vi "play-with-variants.vi"() -> ()   [LabVIEW 2019]
uses:
  <vilib>/Utility/Data Type/Type Definitions/Data Type.ctl
  <vilib>/Utility/Data Type/Type Definitions/Type Definition Info.ctl
  <vilib>/Rock Robotics/WPI/ThirdParty/JAS_Junk/TrajLib/SIMPLE_MOTOR_FF.ctl
  <vilib>/Rock Robotics/WPI/ThirdParty/JAS_Junk/TrajLib/MECA_DRIVE_KINEMATICS.ctl
  <vilib>/Rock Robotics/WPI/ThirdParty/JAS_Junk/TrajLib/TRANSLATION2D.ctl
  <vilib>/Analysis/Matrix/Datatypes/RealMatrix.ctl
  <vilib>/Rock Robotics/WPI/ThirdParty/JAS_Junk/TrajLib/SWERVE_DRIVE_KINEMATICS.ctl
  <vilib>/Rock Robotics/SystemInterfaces/NetworkCommunication/NetComm_UsageReport_report.vi
  <vilib>/Rock Robotics/WPI/ThirdParty/JAS_Junk/TrajLib/Util_LibraryGlobals.vi
  <vilib>/Rock Robotics/WPI/ThirdParty/JAS_Junk/TrajLib/Trajectory_Library.lvlib
  <vilib>/Analysis/Matrix/NI_Matrix.lvlib
  <vilib>/Utility/Data Type/NI_Data Type.lvlib
panel:
  out "TypeDefInfo":T1[](array[typedef])
  out "TypeDef":bool[](array[boolean])
  out "Name":string[](array[string])
  out "Type":T2[](array[typedef])
  out "output array":variant[](array[variant])
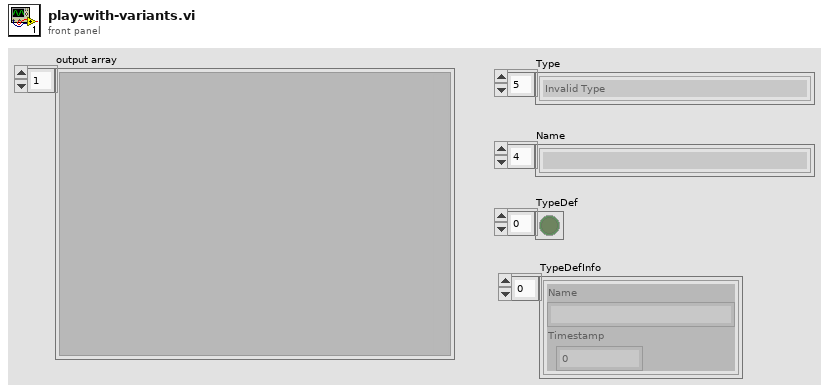
[diagram p1: front panel]
types:
  T1 = typedef "NI_Data Type.lvlib/Type Definition Info.ctl" = cluster{"Name":string, "Timestamp":u32}
  T2 = typedef "NI_Data Type.lvlib/Data Type.ctl" = enum8{"Invalid Type", "Void", "I8", "I16", "I32", "I64", "U8", "U16", "U32", "U64", "Single Float", "Double Float", "Extended Float", "Single Complex", "Double Complex", "Extended Complex", "Enum U8", "Enum U16", "Enum U32", "Enum U64", "Single Float With Unit", "Double Float With Unit", "Extended Float With Unit", "Single Complex with Unit", "Double Complex with Unit", "Extended Complex with Unit", "Boolean", "String", "Path", "Picture", "Tag", "Array", "Cluster", "Variant", "LV Variant", "Waveform", "Timestamp", "Digital Waveform", "Digital Data", "ExpressData", "Refnum", "External Data", "VI", "Poly VI", "LabVIEW Class Instance", "Fixed Point", "Set Collection", "Map Collection"}
  T3 = typedef "Trajectory_Library.lvlib/SWERVE_DRIVE_KINEMATICS.ctl" = cluster{"NumModules":i32, "InverseKinematics":T4, "ForwardKinematics":T4, "Modules":T5[], "PrevCoR":T5}
  T4 = typedef "NI_Matrix.lvlib/RealMatrix.ctl" = dbl[][]
  T5 = typedef "Trajectory_Library.lvlib/TRANSLATION2D.ctl" = cluster{"X":dbl, "Y":dbl}
  T6 = typedef "Trajectory_Library.lvlib/MECA_DRIVE_KINEMATICS.ctl" = cluster{"FrontLeft":T5, "FrontRight":T5, "RearLeft":T5, "RearRight":T5, "InverseKinematics":T4, "ForwardKinematics":T4, "PrevCoR":T5}
  T7 = typedef "Trajectory_Library.lvlib/SIMPLE_MOTOR_FF.ctl" = cluster{"Ks":dbl, "Kv":dbl, "Ka":dbl}
  T8 = typedef "Trajectory_Library.lvlib/DIFF_DRIVE_KINEMATICS.ctl" = cluster{"TrackWidth_Meters":dbl}
  T9 = typedef "Trajectory_Library.lvlib/TRAJ_CONSTRAINT_MECA_DRIVE_KINEMATICS.ctl" = cluster{"Max Speed (M/S)":dbl, "MECA_DRIVE_KINEMATICS":T6}
  T10 = typedef "Trajectory_Library.lvlib/TRAJ_CONSTRAINT_SWERVE_DRIVE_KINEMATICS.ctl" = cluster{"Max Speed (M/S)":dbl, "SwerveKinematics":T3}
  T11 = typedef "Trajectory_Library.lvlib/TRAJ_CONSTRAINT_DIIF_DRIVE_VOLTAGE.ctl" = cluster{"Max Voltage":dbl, "DIFF_DRIVE_KINEMATICS":T8, "SIMPLE_MOTOR_FF":T7}
  T12 = typedef "Trajectory_Library.lvlib/TRAJ_CONSTRAINT_CENTRIPETAL_ACCEL.ctl" = cluster{"Max Cent Accel":dbl}
  T13 = typedef "Trajectory_Library.lvlib/TRAJ_CONSTRAINT_DIIF_DRIVE_KINEMATICS.ctl" = cluster{"Max Speed (M/S)":dbl, "DIFF_DRIVE_KINEMATICS":T8}
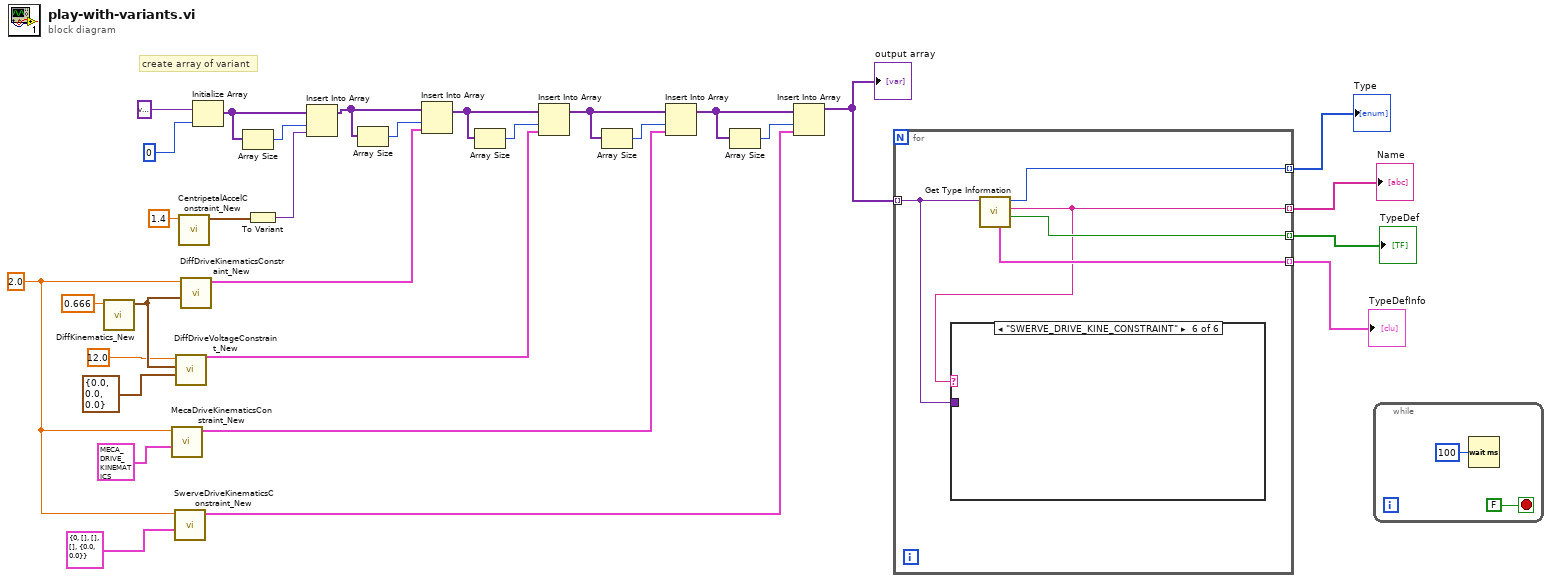
[diagram p0: block diagram]
diagram:
  w12 = 2.0 ("Max Speed (M/S)")
  # "create array of variant"
  n1 = call <vilib>:"DiffKinematics_New.vi"("TrackWidth_Meters"=0.666) -> ("DIFF_DRIVE_KINEMATICS"=w13:T8)  [unwired: 10 in]
  n2 = call <vilib>:"MecaDriveKinematicsConstraint_New.vi"("MecanumKinematics"=T6 {"FrontLeft"={"X"=0.0, "Y"=0.0}, "FrontRight"={"X"=0.0, "Y"=0.0}, "RearLeft"={"X"=0.0, "Y"=0.0}, "RearRight"={"X"=0.0, "Y"=0.0}, "InverseKinematics"=[[0.0, 1.0, -1.0, 0.0], [0.0, 1.0, 1.0, 0.0], [0.0, 1.0, 1.0, 0.0], [0.0, 1.0, -1.0, 0.0]], "ForwardKinematics"=[[0.0, 1.0, -1.0, 0.0], [0.0, 1.0, 1.0, 0.0], [0.0, 1.0, 1.0, 0.0], [0.0, 1.0, -1.0, 0.0]], "PrevCoR"={"X"=0.0, "Y"=0.0}}, "Max Speed (M/S)"=w12) -> ("MECANUM_DRIVE_KINE_CONSTRAINT"=w17:T9)  [unwired: 9 in]
  n3 = call <vilib>:"SwerveDriveKinematicsConstraint_New.vi"("SwerveKinematics"=T3 {"NumModules"=0, "InverseKinematics"=[], "ForwardKinematics"=[], "Modules"=[], "PrevCoR"={"X"=0.0, "Y"=0.0}}, "Max Speed (M/S)"=w12) -> ("SWERVE_DRIVE_KINE_CONSTRAINT"=w16:T10)  [unwired: 9 in]
  n4 = call <vilib>:"DiffDriveVoltageConstraint_New.vi"("SIMPLE_MOTOR_FF"=T7 {"Ks"=0.0, "Kv"=0.0, "Ka"=0.0}, "DIFF_DRIVE_KINEMATICS"=w13, "Max Voltage"=12.0) -> ("DIFF_DRIVE_VOLTAGE_CONSTRAINT"=w18:T11)  [unwired: 8 in]
  n5 = call <vilib>:"CentripetalAccelConstraint_New.vi"("Max Cent Accel"=1.4) -> ("CENTRIPETAL_ACCEL_CONSTRAINT"=w2:T12)  [unwired: 10 in]
  n6 = call <vilib>:"DiffDriveKinematicsConstraint_New.vi"("DIFF_DRIVE_KINEMATICS"=w13, "Max Speed (M/S)"=w12) -> ("DIFF_DRIVE_KINE_CONSTRAINT"=w19:T13)  [unwired: 9 in]
  n7 = Initialize Array(variant, 0 ("dimension size")) -> (w29:variant[])
  n8 = Array Size(array=w29) -> (size(s)=w28:i32)
  n9 = To Variant(anything=w2) -> (Variant=w1:variant)
  n10 = Insert Into Array(array=w29, index=w28, new element=w1) -> (w23:variant[])
  n11 = Array Size(array=w23) -> (size(s)=w27:i32)
  n12 = Insert Into Array(array=w23, index=w27, new element=w19) -> (w22:variant[])
  n13 = Array Size(array=w22) -> (size(s)=w26:i32)
  n14 = Insert Into Array(array=w22, index=w26, new element=w18) -> (w21:variant[])
  n15 = Array Size(array=w21) -> (size(s)=w25:i32)
  n16 = Insert Into Array(array=w21, index=w25, new element=w17) -> (w20:variant[])
  n17 = Array Size(array=w20) -> (size(s)=w24:i32)
  n18 = Insert Into Array(array=w20, index=w24, new element=w16) -> (w7:variant[])
  "output array" <- w7
  n19 = for {
    tunnel: w7 -> [w32] mode=indexing
    tunnel: [w36] -> w6 mode=indexing
    tunnel: [w33] -> w5 mode=indexing
    tunnel: [w34] -> w4 mode=indexing
    tunnel: [w35] -> w3 mode=indexing
    n20 = call <vilib>:"Get Type Information.vi"("variant"=w32) -> ("type definition"=w34:bool, "name"=w33:string, "type"=w36:T2, "type definition info"=w35:T1)  [unwired: 6 in, 1 out]
    n21 = case shown="\"SWERVE_DRIVE_KINE_CONSTRAINT\"" w33 {
      tunnel: w32 -> [_ _ _ _ _ _]
      frame Default {
      }
      frame "DIFF_DRIVE_KINE_CONSTRAINT" {
      }
      frame "CENTRIPETAL_ACCEL_CONSTRAINT" {
      }
      frame "DIFF_DRIVE_VOLTAGE_CONSTRAINT" {
      }
      frame "MECANUM_DRIVE_KINE_CONSTRAINT" {
      }
      frame "SWERVE_DRIVE_KINE_CONSTRAINT" {
      }
    }
  }
  "Type" <- w6
  "Name" <- w5
  "TypeDef" <- w4
  "TypeDefInfo" <- w3
  n22 = while {
    stop <- FALSE stop-if-true
    n23 = Wait (ms)(milliseconds to wait=u32 100) -> ()  [unwired: 1 out]
  }
